vi "C4Hdl_getDiaphusLocation.vi"(0 "c4hdl in":refnum<k24>, 11 "error in (no error)":errorcluster) -> (4 "c4hdl out":refnum<k24>, 6 "diaphusLocation out":string, 15 "error out":errorcluster)   [LabVIEW 2015, in "libC4HdlLV.lvlib"]
uses:
  libC4HdlLV.lvlib
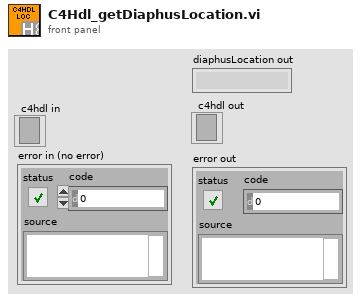
[diagram p1: front panel]
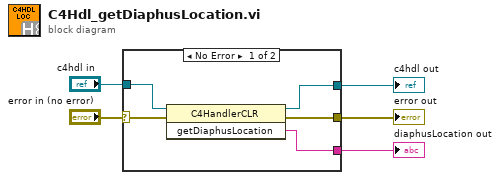
[diagram p0: block diagram]
diagram:
  n1 = case shown="No Error" "error in (no error)" {
    selector: "error in (no error)" -> [w8 w12]
    tunnel: [w10 w12] -> w5
    tunnel: [w9 w11] -> w4
    tunnel: "c4hdl in" -> [w7 w11]
    tunnel: [w6 _] -> w1
    frame No Error {
      n2 = invoke class="C4HandlerCLR" method="getDiaphusLocation"(reference=w7, error in=w8) -> (reference out=w9:refnum<k24>, error out=w10:errorcluster, "getDiaphusLocation"=w6:string)  [unwired: 1 in]
    }
    frame Error {
    }
  }
  "error out" <- w5
  "c4hdl out" <- w4
  "diaphusLocation out" <- w1
